vi "Add Point.vi"(8 "error in (no error)":errorcluster, 9 "Y":dbl, 10 "X":dbl, 11 "IV_data in":refnum<class "IV_data.lvclass">) -> (0 "error out":errorcluster, 3 "IV_data out":refnum<class "IV_data.lvclass">)   [LabVIEW 2018, in "IV_data.lvclass"]
uses:
  IV_data.lvclass
  IV_data.lvclass/IV_data.ctl
  Abstract/Data/Data2D/Data2D.lvclass
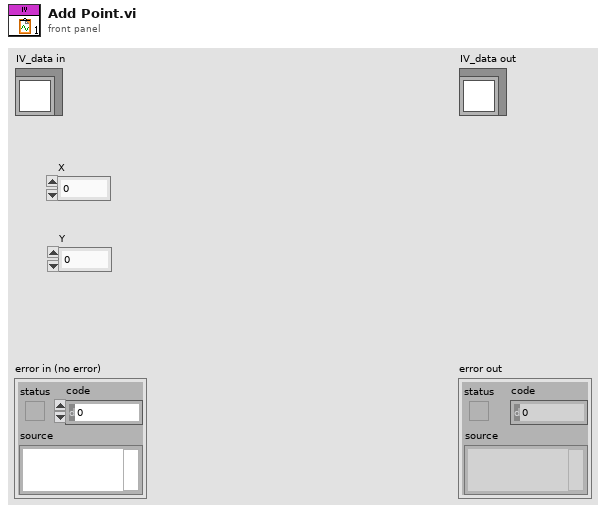
[diagram p1: front panel]
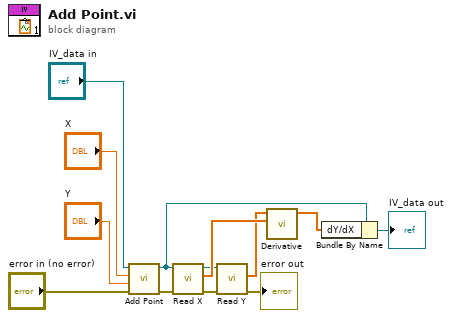
[diagram p0: block diagram]
diagram:
  n1 = call-parent "Add Point.vi"("error in (no error)"="error in (no error)", "Y"="Y", "X"="X", "Data2D in"="IV_data in") -> ("error out"=w2:errorcluster, "Data2D out"=w7:refnum<class "IV_data.lvclass">)  [unwired: 6 in]
  n2 = call-dynamic "Read X.vi"("error in (no error)"=w2, "IV_data in"=w7) -> ("error out"=w3:errorcluster, "X"=w6:dbl[], "IV_data out"=w5:refnum<class "IV_data.lvclass">)  [unwired: 7 in]
  n3 = call-dynamic "Read Y.vi"("error in (no error)"=w3, "IV_data in"=w5) -> ("error out"=→"error out":errorcluster, "Y"=w4:dbl[])  [unwired: 7 in, 1 out]
  n4 = call "Derivative.vi"("X"=w6, "Y"=w4) -> ("dY/dX"=w9:dbl[])  [unwired: 9 in]
  n5 = Bundle By Name(cluster=w7, "dY/dX"=w9) -> (→"IV_data out":refnum<class "IV_data.lvclass">)
